vi "Subvi Write Metadata.vi"(0 "YOffsetIn":i32, 1 "XOffsetIn":i32, 2 "Next Cut":u32, 3 "Store Offset (F)":bool, 4 "TileXYCoordinates":i32[][](array[numeric]), 5 "UserFields":T1, 6 "ROIListBoxIn":string[][](array[string]), 7 "Update (F)":bool) -> ()   [LabVIEW 2012]
uses:
  ProSCI Global.vi
  ProSCI ConfigGlobal.vi
  <vilib>/Utility/config.llb/Write Key (String).vi
  <vilib>/Utility/config.llb/Write Key (U32).vi
  <vilib>/Utility/config.llb/Write Key (I32).vi
  <vilib>/Utility/config.llb/NI_LVConfig.lvlib
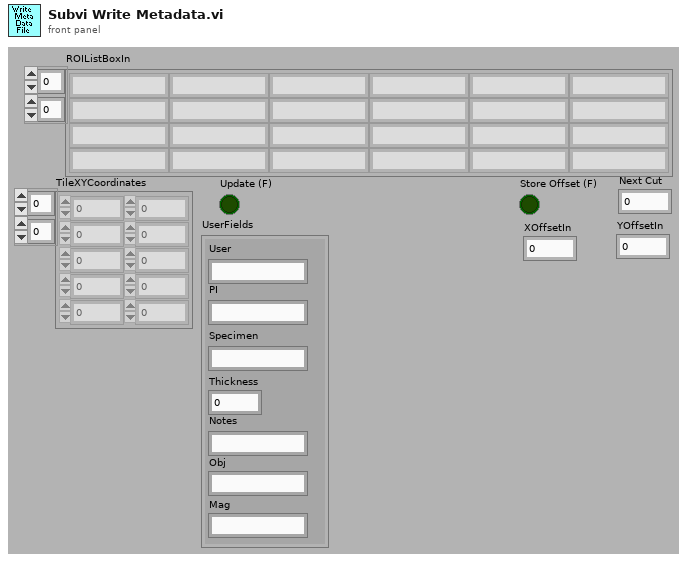
[diagram p1: front panel]
types:
  T1 = cluster{"User":string, "PI":string, "Specimen":string, "Thickness":u16, "Notes":string, "Obj":string, "Mag":string}
  T2 = typedef "NI_LVConfig.lvlib/Config Data RefNum.ctl" = refnum<k1>
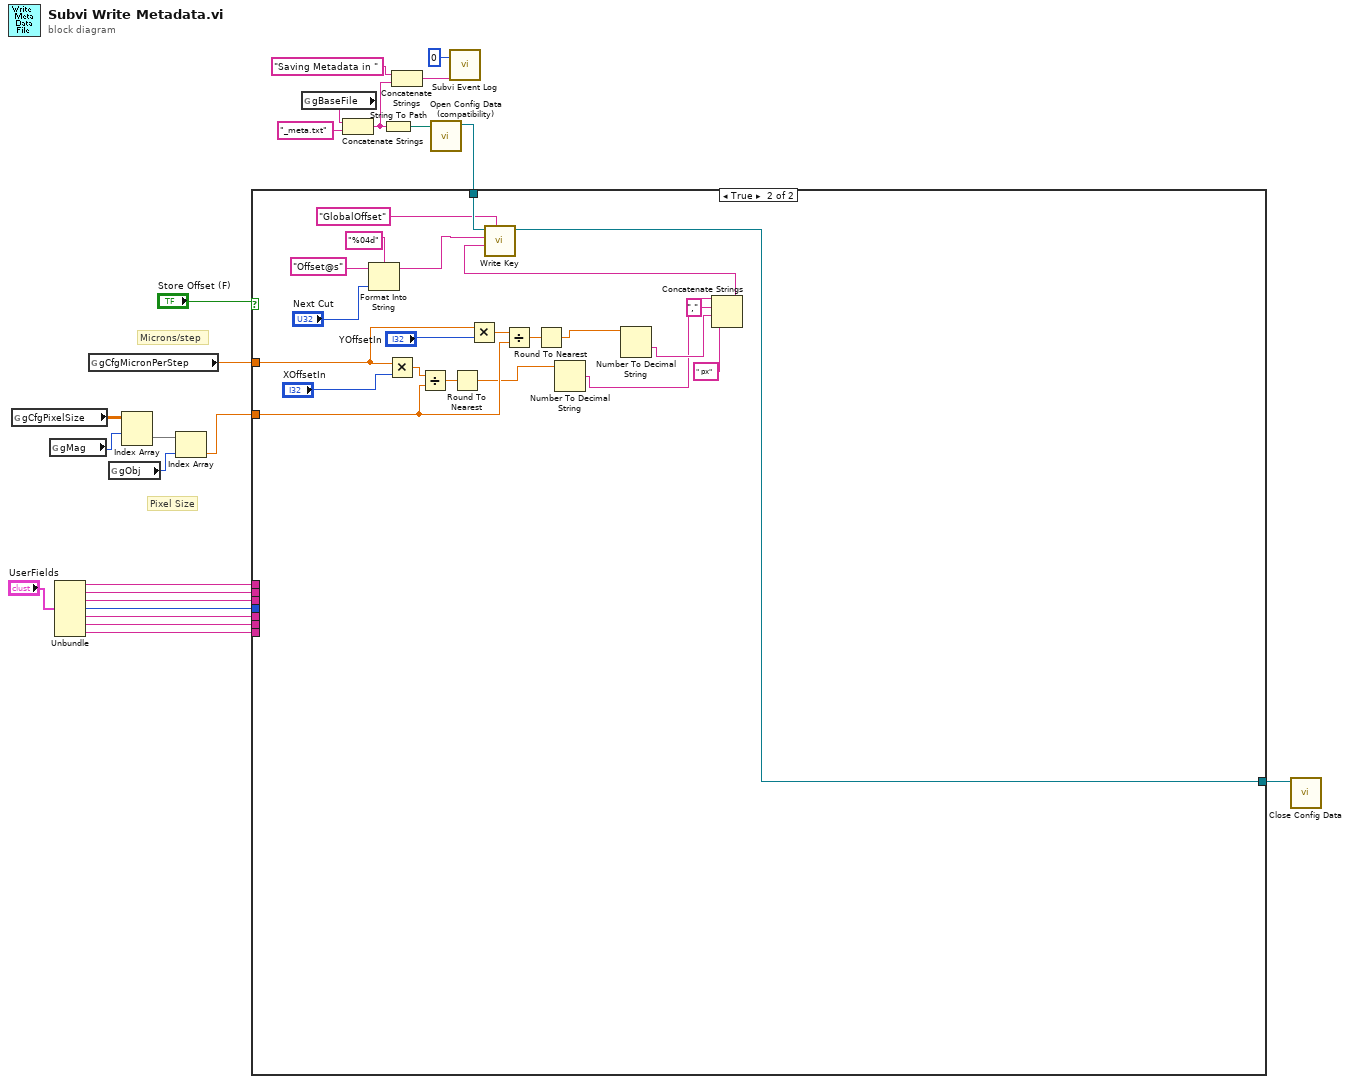
[diagram p0: block diagram]
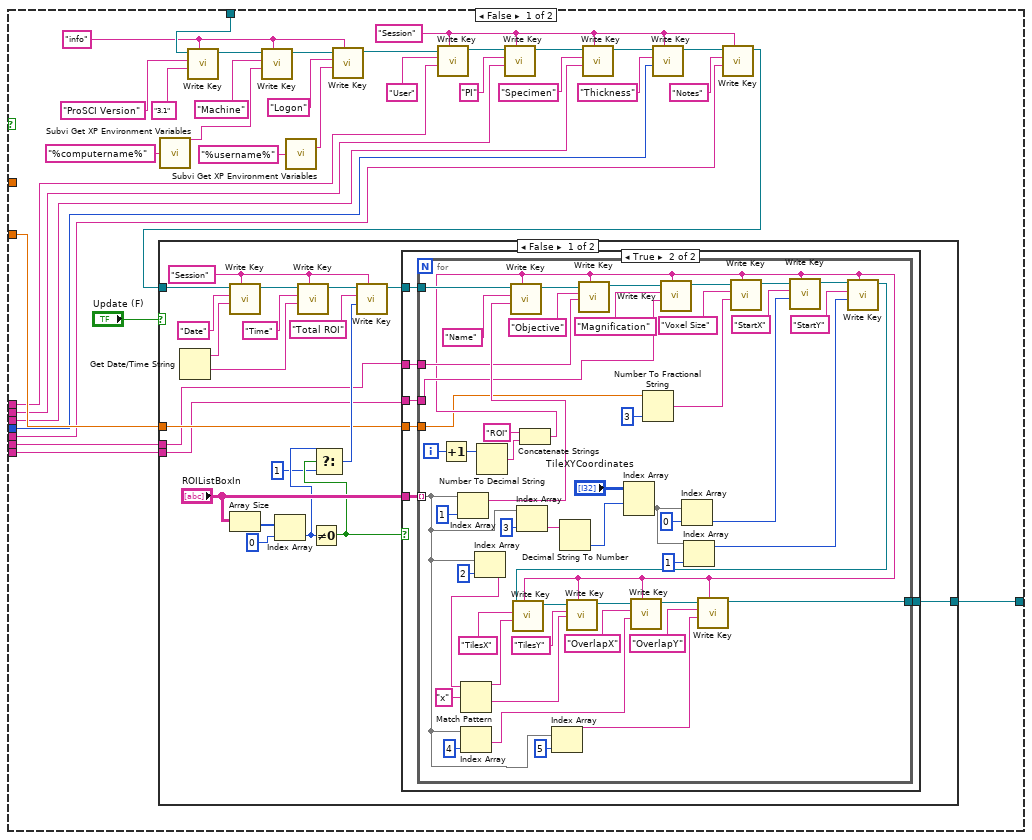
[diagram p2: hidden frame]
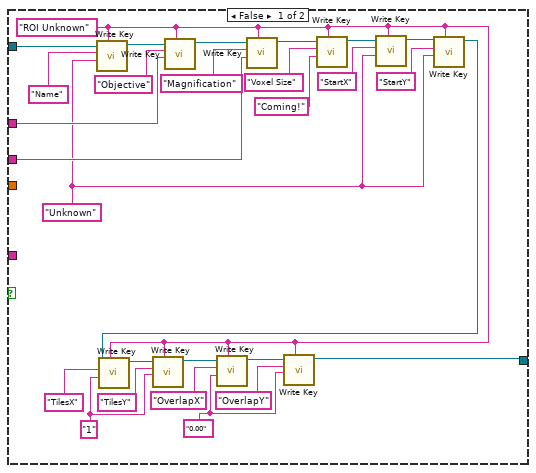
[diagram p3: hidden frame]
diagram:
  # "Pixel Size"
  # "Microns/step"
  n1 = global read "ProSCI ConfigGlobal.vi" "gCfgPixelSize"() -> (w15:dbl[][])
  n2 = global read "ProSCI Global.vi" "gMag"() -> (w14:u8)
  n3 = Unbundle("UserFields") -> ("User"=w7:string, "PI"=w6:string, "Specimen"=w5:string, "Thickness"=w4:u16, "Notes"=w3:string, "Obj"=w2:string, "Mag"=w1:string)
  n4 = global read "ProSCI ConfigGlobal.vi" "gCfgMicronPerStep"() -> (w11:dbl)
  n5 = global read "ProSCI Global.vi" "gObj"() -> (w12:u8)
  n6 = Index Array(array=w15, index (row)=w14) -> (element=w13:dbl[])  [unwired: 1 in]
  n7 = Index Array(array=w13, index=w12) -> (element=w10:dbl)
  n8 = global read "ProSCI Global.vi" "gBaseFile"() -> (w24:string)
  n9 = Concatenate Strings(w24, "_meta.txt" ("string")) -> (w18:string)
  n10 = String To Path(string=w18) -> (path=w22:path)
  n11 = Concatenate Strings("Saving Metadata in " ("string"), w18) -> (w17:string)
  n12 = call <vilib>:"Open Config Data (compatibility).vi"("configuration file path"=w22) -> ("refnum"=w21:T2)  [unwired: 8 in, 2 out]
  n13 = case shown="True" "Store Offset (F)" {
    tunnel: w21 -> [w52 w188]
    tunnel: w11 -> [_ w179]
    tunnel: w10 -> [w33 w176]
    tunnel: [w32 w169] -> w9
    tunnel: w7 -> [w31 _]
    tunnel: w6 -> [w30 _]
    tunnel: w5 -> [w29 _]
    tunnel: w4 -> [w28 _]
    tunnel: w3 -> [w27 _]
    tunnel: w2 -> [w26 _]
    tunnel: w1 -> [w25 _]
    frame False {
      w36 = "Session" ("string")
      w51 = "info" ("string")
      n14 = call "Subvi Get XP Environment Variables.vi"("Environment Variable"="%computername%") -> ("Value"=w53:string)  [unwired: 1 out]
      n15 = call-poly <vilib>:"Write Key.vi"("section"=w51, "value"="3.1" ("string"), "key"="ProSCI Version" ("string"), "refnum"=w52) -> ("refnum out"=w48:T2)  [unwired: 2 in, 5 out]
      n16 = call-poly <vilib>:"Write Key.vi"("section"=w51, "value"=w53, "key"="Machine" ("string"), "refnum"=w48) -> ("refnum out"=w47:T2)  [unwired: 2 in, 5 out]
      n17 = call "Subvi Get XP Environment Variables.vi"("Environment Variable"="%username%") -> ("Value"=w49:string)  [unwired: 1 out]
      n18 = call-poly <vilib>:"Write Key.vi"("section"=w51, "value"=w49, "key"="Logon" ("string"), "refnum"=w47) -> ("refnum out"=w46:T2)  [unwired: 2 in, 5 out]
      n19 = call-poly <vilib>:"Write Key.vi"("section"=w36, "value"=w31, "key"="User" ("string"), "refnum"=w46) -> ("refnum out"=w45:T2)  [unwired: 2 in, 5 out]
      n20 = call-poly <vilib>:"Write Key.vi"("section"=w36, "value"=w30, "key"="PI" ("string"), "refnum"=w45) -> ("refnum out"=w44:T2)  [unwired: 2 in, 5 out]
      n21 = call-poly <vilib>:"Write Key.vi"("section"=w36, "value"=w29, "key"="Specimen" ("string"), "refnum"=w44) -> ("refnum out"=w43:T2)  [unwired: 2 in, 5 out]
      n22 = call-poly <vilib>:"Write Key.vi"("section"=w36, "value"=w28, "key"="Thickness" ("string"), "refnum"=w43) -> ("refnum out"=w42:T2)  [unwired: 1 in, 6 out]
      n23 = call-poly <vilib>:"Write Key.vi"("section"=w36, "value"=w27, "key"="Notes" ("string"), "refnum"=w42) -> ("refnum out"=w34:T2)  [unwired: 2 in, 5 out]
      n24 = case shown="False" "Update (F)" {
        tunnel: w34 -> [w74 w166]
        tunnel: [w73 w166] -> w32
        tunnel: w33 -> [w61 _]
        tunnel: w26 -> [w60 _]
        tunnel: w25 -> [w59 _]
        frame False {
          w69 = "Session" ("string")
          n25 = Get Date/Time String() -> (date string=w76:string, time string=w75:string)  [unwired: 3 out]
          n26 = call-poly <vilib>:"Write Key.vi"("section"=w69, "value"=w76, "key"="Date" ("string"), "refnum"=w74) -> ("refnum out"=w79:T2)  [unwired: 2 in, 5 out]
          n27 = Array Size(array="ROIListBoxIn") -> (size(s)=w71:i32[])
          n28 = Index Array(array=w71, index=0) -> (element=w64:i32)
          n29 = call-poly <vilib>:"Write Key.vi"("section"=w69, "value"=w75, "key"="Time" ("string"), "refnum"=w79) -> ("refnum out"=w68:T2)  [unwired: 2 in, 5 out]
          n30 = Not Equal To 0?(x=w64) -> (x != 0?=w65:bool)
          n31 = Select(t=w64, s=w65, f=1) -> (s? t:f=w62:i32)
          n32 = call-poly <vilib>:"Write Key.vi"("section"=w69, "value"=w62, "key"="Total ROI" ("string"), "refnum"=w68) -> ("refnum out"=w67:T2)  [unwired: 1 in, 6 out]
          n33 = case shown="True" w65 {
            tunnel: w67 -> [w107 w113]
            tunnel: w60 -> [w90 w112]
            tunnel: w59 -> [w89 w111]
            tunnel: [w98 w110] -> w73
            tunnel: "ROIListBoxIn" -> [_ w109]
            tunnel: w61 -> [_ w108]
            frame False {
              w80 = "0.00" ("string")
              w81 = "1" ("string")
              w82 = "Unknown" ("string")
              w83 = "ROI Unknown" ("string")
              n34 = call-poly <vilib>:"Write Key.vi"("section"=w83, "value"=w82, "key"="Name" ("string"), "refnum"=w107) -> ("refnum out"=w106:T2)  [unwired: 2 in, 5 out]
              n35 = call-poly <vilib>:"Write Key.vi"("section"=w83, "value"=w90, "key"="Objective" ("string"), "refnum"=w106) -> ("refnum out"=w105:T2)  [unwired: 2 in, 5 out]
              n36 = call-poly <vilib>:"Write Key.vi"("section"=w83, "value"=w89, "key"="Magnification" ("string"), "refnum"=w105) -> ("refnum out"=w104:T2)  [unwired: 2 in, 5 out]
              n37 = call-poly <vilib>:"Write Key.vi"("section"=w83, "value"="Coming!" ("string"), "key"="Voxel Size" ("string"), "refnum"=w104) -> ("refnum out"=w103:T2)  [unwired: 2 in, 5 out]
              n38 = call-poly <vilib>:"Write Key.vi"("section"=w83, "value"=w82, "key"="StartX" ("string"), "refnum"=w103) -> ("refnum out"=w102:T2)  [unwired: 2 in, 5 out]
              n39 = call-poly <vilib>:"Write Key.vi"("section"=w83, "value"=w82, "key"="StartY" ("string"), "refnum"=w102) -> ("refnum out"=w84:T2)  [unwired: 2 in, 5 out]
              n40 = call-poly <vilib>:"Write Key.vi"("section"=w83, "value"=w81, "key"="TilesX" ("string"), "refnum"=w84) -> ("refnum out"=w101:T2)  [unwired: 2 in, 5 out]
              n41 = call-poly <vilib>:"Write Key.vi"("section"=w83, "value"=w81, "key"="TilesY" ("string"), "refnum"=w101) -> ("refnum out"=w100:T2)  [unwired: 2 in, 5 out]
              n42 = call-poly <vilib>:"Write Key.vi"("section"=w83, "value"=w80, "key"="OverlapX" ("string"), "refnum"=w100) -> ("refnum out"=w99:T2)  [unwired: 2 in, 5 out]
              n43 = call-poly <vilib>:"Write Key.vi"("section"=w83, "value"=w80, "key"="OverlapY" ("string"), "refnum"=w99) -> ("refnum out"=w98:T2)  [unwired: 2 in, 5 out]
            }
            frame True {
              n44 = for {
                tunnel: w109 -> [w128] mode=indexing
                tunnel: w113 -> [w160]
                tunnel: w112 -> [w139]
                tunnel: w111 -> [w138]
                tunnel: [w121] -> w110
                tunnel: w108 -> [w116]
                i -> [w164]
                n45 = Increment(x=w164) -> (x+1=w163:i32)
                n46 = Index Array(array=w128, index=1) -> (element=w158:string)
                n47 = Index Array(array=w128, index=4) -> (element=w123:string)
                n48 = Index Array(array=w128, index=2) -> (element=w135:string)
                n49 = Match Pattern(string=w135, regular expression="x") -> (before substring=w131:string, after substring=w130:string)  [unwired: 3 out]
                n50 = Number To Decimal String(number=w163) -> (decimal integer string=w162:string)  [unwired: 1 out]
                n51 = Index Array(array=w128, index=3) -> (element=w150:string)
                n52 = Concatenate Strings("ROI" ("string"), w162) -> (w120:string)
                n53 = call-poly <vilib>:"Write Key.vi"("section"=w120, "value"=w158, "key"="Name" ("string"), "refnum"=w160) -> ("refnum out"=w157:T2)  [unwired: 2 in, 5 out]
                n54 = Index Array(array=w128, index=5) -> (element=w122:string)
                n55 = Decimal String To Number(string=w150) -> (number=w148:i32)  [unwired: 3 out]
                n56 = call-poly <vilib>:"Write Key.vi"("section"=w120, "value"=w139, "key"="Objective" ("string"), "refnum"=w157) -> ("refnum out"=w156:T2)  [unwired: 2 in, 5 out]
                n57 = Index Array(array="TileXYCoordinates", index (row)=w148) -> (element=w146:i32[])  [unwired: 1 in]
                n58 = Number To Fractional String(number=w116, precision (6)=i16 3) -> (F-format string=w114:string)  [unwired: 2 out]
                n59 = call-poly <vilib>:"Write Key.vi"("section"=w120, "value"=w138, "key"="Magnification" ("string"), "refnum"=w156) -> ("refnum out"=w153:T2)  [unwired: 2 in, 5 out]
                n60 = Index Array(array=w146, index=0) -> (element=w141:i32)
                n61 = Index Array(array=w146, index=1) -> (element=w140:i32)
                n62 = call-poly <vilib>:"Write Key.vi"("section"=w120, "value"=w114, "key"="Voxel Size" ("string"), "refnum"=w153) -> ("refnum out"=w145:T2)  [unwired: 2 in, 5 out]
                n63 = call-poly <vilib>:"Write Key.vi"("section"=w120, "value"=w141, "key"="StartX" ("string"), "refnum"=w145) -> ("refnum out"=w144:T2)  [unwired: 1 in, 6 out]
                n64 = call-poly <vilib>:"Write Key.vi"("section"=w120, "value"=w140, "key"="StartY" ("string"), "refnum"=w144) -> ("refnum out"=w137:T2)  [unwired: 1 in, 6 out]
                n65 = call-poly <vilib>:"Write Key.vi"("section"=w120, "value"=w131, "key"="TilesX" ("string"), "refnum"=w137) -> ("refnum out"=w129:T2)  [unwired: 2 in, 5 out]
                n66 = call-poly <vilib>:"Write Key.vi"("section"=w120, "value"=w130, "key"="TilesY" ("string"), "refnum"=w129) -> ("refnum out"=w127:T2)  [unwired: 2 in, 5 out]
                n67 = call-poly <vilib>:"Write Key.vi"("section"=w120, "value"=w123, "key"="OverlapX" ("string"), "refnum"=w127) -> ("refnum out"=w125:T2)  [unwired: 2 in, 5 out]
                n68 = call-poly <vilib>:"Write Key.vi"("section"=w120, "value"=w122, "key"="OverlapY" ("string"), "refnum"=w125) -> ("refnum out"=w121:T2)  [unwired: 2 in, 5 out]
              }
            }
          }
        }
        frame True {
        }
      }
    }
    frame True {
      n69 = Format Into String(format string="%04d", initial string="Offset@s" ("string"), "Next Cut") -> (resulting string=w183:string)  [unwired: 1 in, 1 out]
      n70 = Multiply(x=w179, y="XOffsetIn") -> (x*y=w178:dbl)
      n71 = Divide(x=w178, y=w176) -> (x/y=w175:dbl)
      n72 = Round To Nearest(number=w175) -> (nearest integer value=w171:dbl)
      n73 = Multiply(x=w179, y="YOffsetIn") -> (x*y=w177:dbl)
      n74 = Divide(x=w177, y=w176) -> (x/y=w174:dbl)
      n75 = Round To Nearest(number=w174) -> (nearest integer value=w173:dbl)
      n76 = Number To Decimal String(number=w171) -> (decimal integer string=w170:string)  [unwired: 1 out]
      n77 = Number To Decimal String(number=w173) -> (decimal integer string=w172:string)  [unwired: 1 out]
      n78 = Concatenate Strings(w170, "," ("string"), w172, " px" ("string")) -> (w180:string)
      n79 = call-poly <vilib>:"Write Key.vi"("section"="GlobalOffset" ("string"), "value"=w180, "key"=w183, "refnum"=w188) -> ("refnum out"=w169:T2)  [unwired: 2 in, 5 out]
    }
  }
  n80 = call "Subvi Event Log.vi"("CustomMessage"=w17, "EventNum"=u32 0) -> ()
  n81 = call <vilib>:"Close Config Data.vi"("refnum"=w9) -> ()  [unwired: 2 in, 9 out]
